vi "4_PSK.vi"() -> ()   [LabVIEW 2013]
uses:
  <vilib>/addons/Modulation/Digital/General/MT Generate PSK System Parameters(M).vi
  <vilib>/addons/Modulation/Digital/General/MT Generate Bits (Galois, PN Order).vi
  <vilib>/addons/Modulation/Digital/General/MT Generate PSK Synchronization Parameters (bit array).vi
  <vilib>/addons/Modulation/Digital/General/MT Format Eye Diagram (complex).vi
  <vilib>/addons/Modulation/niDMT.lvlib
panel:
  out "Sync Found Index":dbl
  out "Error Out":errorcluster
  in  "Stop":bool
  out "Measurements":T1
  in  "Eb/N0 (dB)":dbl(slide)=50.0 scale=-10.0..50.0
  in  "Message Bits":i32=100
  in  "M-PSK (4)":i32=4
  out "Output Bitstream":bool[](array[boolean])
  out "Input Bitstream":bool[](array[boolean])
  out "Baseband Waveform":cluster{"t0":dbl, "dt":dbl, "Y":dbl[]}(graph)
  in  "Tab Control":enum32{"Constellation", "Eye Diagram"}(tab)
  out "Constellation Plot":T2(graph)
  out "Eye Diagram":cluster{"t0":dbl, "dt":dbl, "Y":dbl[]}[](graph)
  # "M-PSK Simulation"
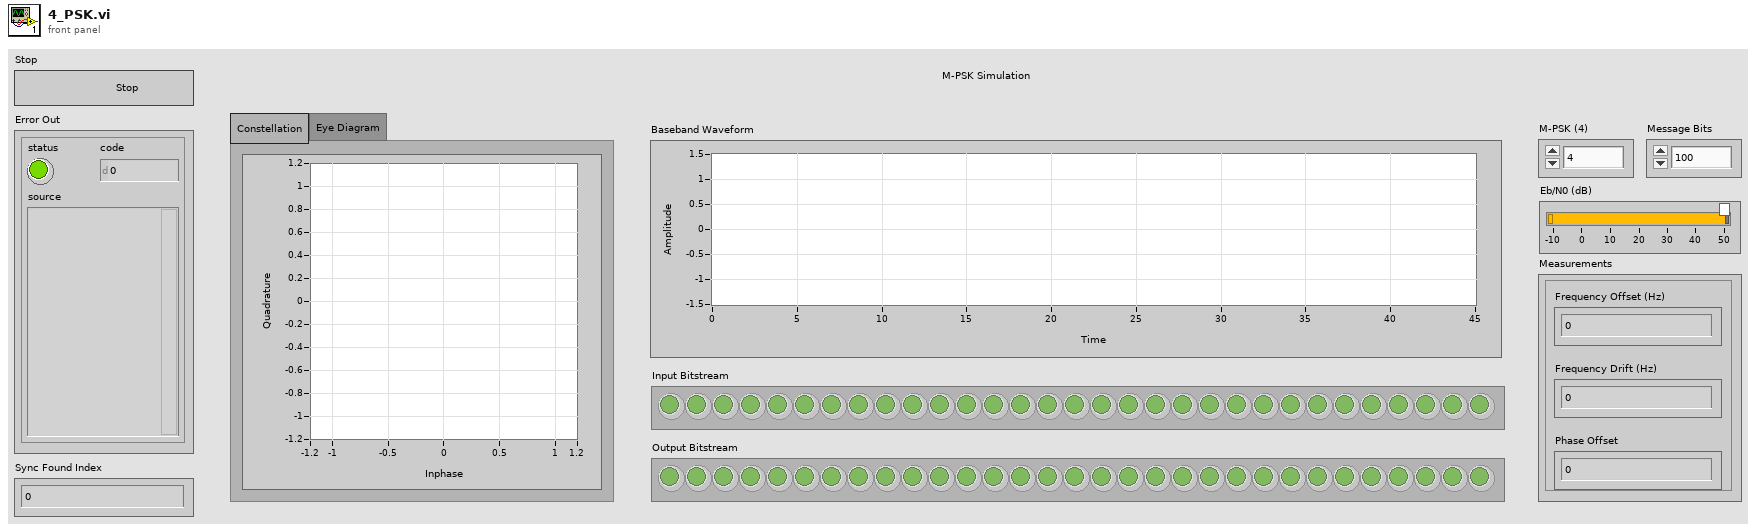
[diagram p1: front panel]
types:
  T1 = cluster{"Frequency Offset (Hz)":dbl, "Frequency Drift (Hz)":dbl, "Phase Offset":dbl}
  T2 = cluster{"constellation":dbl[], "oversampled data":dbl[]}[]
  T3 = enum16{"FSK", "PSK", "QAM", "MSK", "PAM", "ASK", "CPM"}
  T4 = enum16{"none", "Raised Cosine", "Root Raised Cos", "Gaussian"}
  T5 = cluster{"samples per symbol (16)":i32, "symbol map":cdb[], "differential PSK":enum16{"disable", "enable"}, "PSK type":u16}
  T6 = typedef "niAMT.lvlib/Complex Data Waveform.ctl" = cluster{"t0":dbl, "dt":dbl, "Y":cdb[]}
  T7 = cluster{"expected sync location (symbols)":i32, "sync sequence":cdb[], "sync location uncertainty (symbols)":i32, "sync indent (symbols)":i32}
  T8 = cluster{"frequency offset (Hz)":dbl, "frequency drift (Hz)":dbl, "phase offset (deg)":dbl}
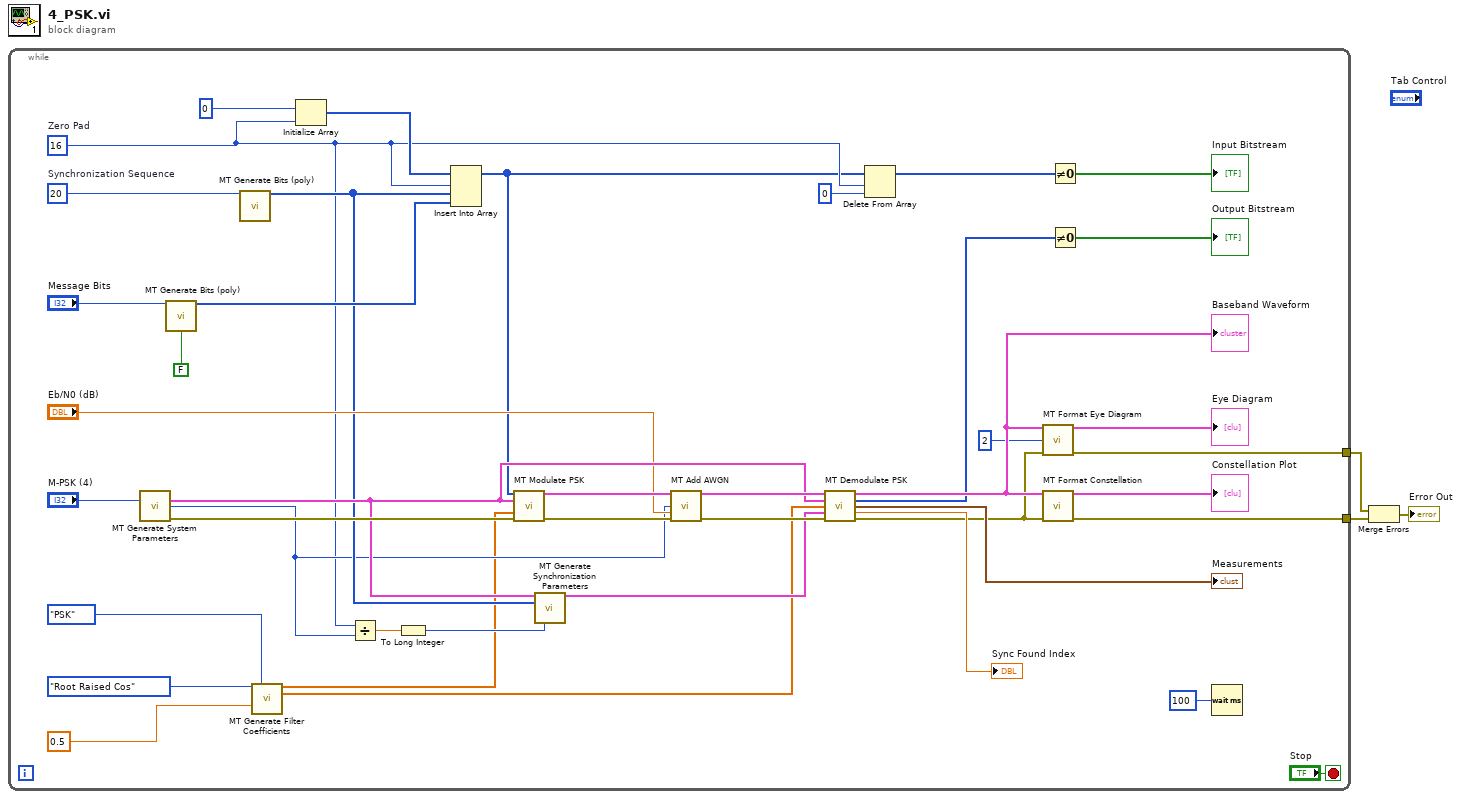
[diagram p0: block diagram]
diagram:
  n1 = while {
    tunnel: [w12] -> w1
    tunnel: [w11] -> w2
    stop <- "Stop" stop-if-true
    w45 = 20  # Synchronization Sequence
    w16 = 16  # Zero Pad
    n2 = call-poly <vilib>:"MT Generate System Parameters.vi"("M-PSK (4)"="M-PSK (4)") -> ("PSK system parameters"=w25:T5, "bits per symbol"=w17:i32, "error out"=w34:errorcluster)  [unwired: 12 in]
    n3 = call-poly <vilib>:"MT Generate Bits (poly).vi"("total bits (128)"="Message Bits", "reset? (T)"=FALSE) -> ("output bit stream"=w23:i8[])  [unwired: 11 in, 2 out]
    n4 = call-poly <vilib>:"MT Generate Bits (poly).vi"("total bits (128)"=w45) -> ("output bit stream"=w18:i8[])  [unwired: 12 in, 2 out]
    n5 = call <vilib>:"MT Generate Filter Coefficients.vi"("pulse shaping filter (none)"=T4."Root Raised Cos", "modulation type"=T3."PSK", "filter parameter"=0.5) -> ("pulse shaping filter coefficients"=w9:dbl[], "matched filter coefficients"=w8:dbl[])  [unwired: 10 in, 1 out]
    n6 = Initialize Array "Initialize Array"(0, w16) -> (w41:i32[])
    n7 = Divide(x=w16, y=w17) -> (x/y=w20:dbl)
    n8 = To Long Integer(number=w20) -> (32bit integer=w19:i32)
    n9 = Insert Into Array "Insert Into Array"(array=w41, index=w16, new element #1=w18, new element #2=w23) -> (w4:i32[])
    n10 = call <vilib>:"MT Modulate PSK.vi"("input bit stream"=w4, "PSK system parameters"=w25, "pulse shaping filter coefficients"=w9, "error in (no error)"=w34) -> ("output complex waveform"=w33:T6, "error out"=w32:errorcluster)  [unwired: 9 in, 1 out]
    n11 = call-poly <vilib>:"MT Generate Synchronization Parameters.vi"("PSK system parameters"=w25, "sync bits"=w18, "expected sync location (symbols)"=w19) -> ("PSK synchronization parameters"=w24:T7)  [unwired: 11 in, 1 out]
    n12 = call <vilib>:"MT Add AWGN.vi"("input complex waveform"=w33, "bits per symbol (1)"=w17, "Eb/N0 (10 dB)"="Eb/N0 (dB)", "error in (no error)"=w32) -> ("output complex waveform"=w30:T6, "error out"=w31:errorcluster)  [unwired: 9 in, 1 out]
    n13 = call <vilib>:"MT Demodulate PSK.vi"("input complex waveform"=w30, "PSK system parameters"=w25, "matched filter coefficients"=w8, "synchronization parameters"=w24, "error in (no error)"=w31) -> ("recovered complex waveform"=w28:T6, "output bit stream"=w14:i8[], "measurements"=→"Measurements":T8, "sync found index (symbols)"=→"Sync Found Index":dbl, "error out"=w10:errorcluster)  [unwired: 6 in]
    "Baseband Waveform" <- w28
    n14 = Delete From Array "Delete From Array"(array=w4, length=w16, index=0) -> (array with subset deleted=w40:i32[])  [unwired: 1 out]
    n15 = call-poly <vilib>:"MT Format Eye Diagram.vi"("waveform"=w28, "eye length"=2, "error in (no error)"=w10) -> ("eye diagram"=→"Eye Diagram":cluster{"t0":dbl, "dt":dbl, "Y":dbl[]}[], "error out"=w12:errorcluster)  [unwired: 11 in]
    n16 = call <vilib>:"MT Format Constellation.vi"("waveform"=w28, "error in (no error)"=w10) -> ("constellation graph"=→"Constellation Plot":T2, "error out"=w11:errorcluster)  [unwired: 12 in]
    n17 = Not Equal To 0?(x=w40) -> (x != 0?=→"Input Bitstream":bool[])
    n18 = Not Equal To 0?(x=w14) -> (x != 0?=→"Output Bitstream":bool[])
    n19 = Wait (ms)(milliseconds to wait=100) -> ()  [unwired: 1 out]
  }
  n20 = Merge Errors(w1, w2) -> (→"Error Out":errorcluster)
